vi "Configure Library in Memory for Development.vi"(7 "target name (My Computer)":string="My Computer", 10 "save VIs? (T)":bool=TRUE, 11 "library name":string="DSF Core.lvlib") -> (0 "error out":errorcluster)   [LabVIEW 2019, in "Build Automation.lvlib"]
uses:
  Build Automation.lvlib
panel:
  in  "enable debug? (F)":bool
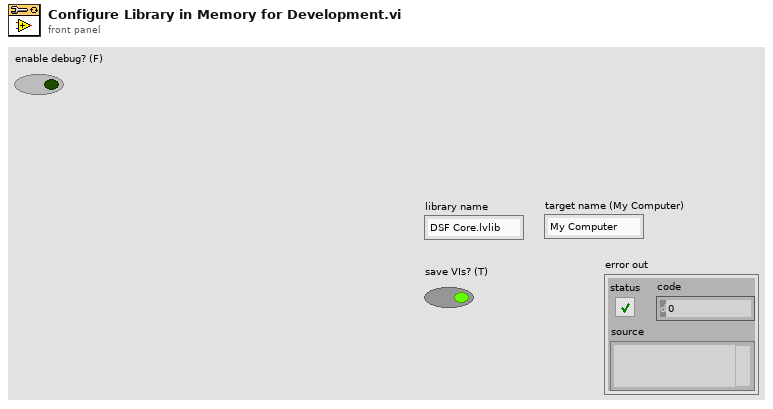
[diagram p1: front panel]
types:
  T1 = enum16{"Share clones between instances", "Preallocate clone for each instance"}
  T2 = cluster{"Status Message":refnum<data-value>, "Progress":refnum<data-value>, "Stop":refnum<data-value>}
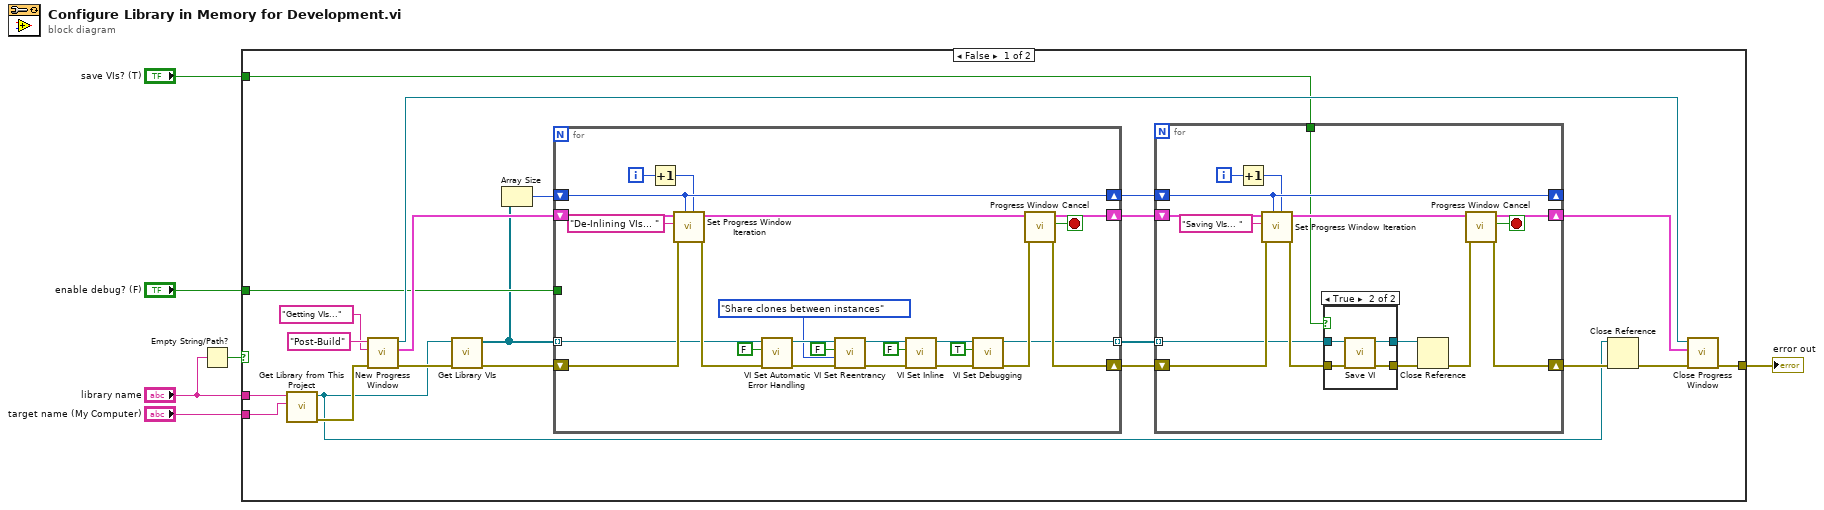
[diagram p0: block diagram]
diagram:
  n1 = Empty String/Path?(string/path="library name") -> (empty?=w5:bool)
  n2 = case shown="False" w5 {
    tunnel: [w25 _] -> w3
    tunnel: "enable debug? (F)" -> [w24 _]
    tunnel: "library name" -> [w13 _]
    tunnel: "save VIs? (T)" -> [w10 _]
    tunnel: "target name (My Computer)" -> [w11 _]
    frame False {
      n3 = call "Get Library from This Project.vi"("Target Name (My Computer)"=w11, "Library Name"=w13) -> ("error out"=w12:errorcluster, "Library Refnum"=w8:refnum<vi>)  [unwired: 8 in]
      n4 = call "New Progress Window.vi"("error in (no error)"=w12, "Initial Message"="Getting VIs...", "Window Title"="Post-Build" ("WindowTitle")) -> ("error out"=w27:errorcluster, "DVRs"=w26:T2, "VI refnum"=w28:refnum<vi>)  [unwired: 6 in]
      n5 = call "Get Library VIs.vi"("error in (no error)"=w27, "library ref"=w8) -> ("error out"=w7:errorcluster, "vi refs"=w22:refnum<vi>[])  [unwired: 8 in]
      n6 = Array Size(array=w22) -> (size(s)=w23:i32)
      n7 = for {
        tunnel: w22 -> [w43] mode=indexing
        shift-right: [w51] -> w20
        shift-left: w26 -> [w48]
        shift-right: [w44] -> w18
        shift-left: w7 -> [w46]
        tunnel: w24 -> [_]
        tunnel: [w32] -> w19 mode=indexing
        shift-right: [w42] -> w21
        shift-left: w23 -> [w42]
        i -> [w53]
        stop <- w52 stop-if-true
        n8 = Increment(x=w53) -> (x+1=w41:i32)
        n9 = call "Set Progress Window Iteration.vi"("current iteration"=w41, "total iterations"=w42, "error in (no error)"=w46, "Status Message"="De-Inlining VIs... ", "DVRs in"=w48) -> ("error out"=w45:errorcluster, "DVRs out"=w47:T2)  [unwired: 5 in]
        n10 = call "VI Set Automatic Error Handling.vi"("error in (no error)"=w45, "Automatic Error Handling"=FALSE, "vi ref in"=w43) -> ("error out"=w31:errorcluster, "vi ref out"=w49:refnum<vi>)  [unwired: 7 in]
        n11 = call "VI Set Reentrancy.vi"("error in (no error)"=w31, "Reentrancy Type (shared clone)"=T1."Share clones between instances", "Is Reentrant"=FALSE, "vi ref in"=w49) -> ("error out"=w36:errorcluster, "vi ref out"=w37:refnum<vi>)  [unwired: 6 in]
        n12 = call "VI Set Inline.vi"("error in (no error)"=w36, "Inline VI"=FALSE, "vi ref in"=w37) -> ("error out"=w34:errorcluster, "vi ref out"=w35:refnum<vi>)  [unwired: 7 in]
        n13 = call "VI Set Debugging.vi"("error in (no error)"=w34, "Allow Debugging"=TRUE, "vi ref in"=w35) -> ("error out"=w33:errorcluster, "vi ref out"=w32:refnum<vi>)  [unwired: 7 in]
        n14 = call "Progress Window Cancel.vi"("error in (no error)"=w33, "DVRs in"=w47) -> ("error out"=w44:errorcluster, "cancelled"=w52:bool, "DVRs out"=w51:T2)  [unwired: 7 in]
      }
      n15 = for {
        tunnel: w19 -> [w55] mode=indexing
        shift-right: [w67] -> w17
        shift-left: w20 -> [w66]
        shift-right: [w63] -> w15
        shift-left: w18 -> [w64]
        shift-right: [w62] -> _
        shift-left: w21 -> [w62]
        tunnel: w10 -> [w54]
        i -> [w69]
        stop <- w68 stop-if-true
        n16 = Increment(x=w69) -> (x+1=w61:i32)
        n17 = call "Set Progress Window Iteration.vi"("current iteration"=w61, "total iterations"=w62, "error in (no error)"=w64, "Status Message"="Saving VIs... ", "DVRs in"=w66) -> ("error out"=w59:errorcluster, "DVRs out"=w65:T2)  [unwired: 5 in]
        n18 = case shown="True" w54 {
          tunnel: w59 -> [w70 w75]
          tunnel: [w71 w74] -> w58
          tunnel: [w70 w73] -> w57
          tunnel: w55 -> [w71 w72]
          frame False {
          }
          frame True {
            n19 = call "Save VI.vi"("error in (no error)"=w75, "vi ref in"=w72) -> ("error out"=w73:errorcluster, "vi ref out"=w74:refnum<vi>)  [unwired: 8 in]
          }
        }
        n20 = Close Reference(reference=w58, error in (no error)=w57) -> (error out=w56:errorcluster)
        n21 = call "Progress Window Cancel.vi"("error in (no error)"=w56, "DVRs in"=w65) -> ("error out"=w63:errorcluster, "cancelled"=w68:bool, "DVRs out"=w67:T2)  [unwired: 7 in]
      }
      n22 = Close Reference(reference=w8, error in (no error)=w15) -> (error out=w14:errorcluster)
      n23 = call "Close Progress Window.vi"("error in (no error)"=w14, "DVRs in"=w17, "VI refnum"=w28) -> ("error out"=w25:errorcluster)  [unwired: 8 in]
    }
    frame True {
    }
  }
  "error out" <- w3
